vi "04.2 Create Invoke Nodes.vi"() -> ()   [LabVIEW 2019]
uses:
  <vilib>/numeric/Random Number (Range) DBL.vi
panel:
  in  "Stop":bool
  out "Waveform Chart":dbl(graph)
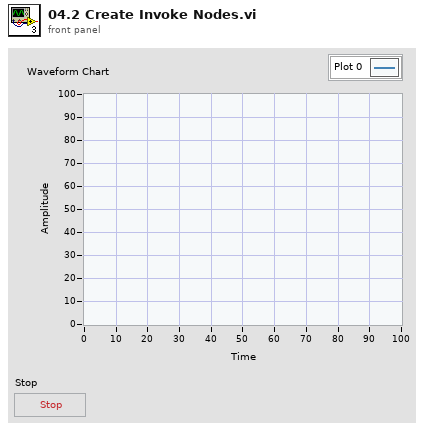
[diagram p1: front panel]
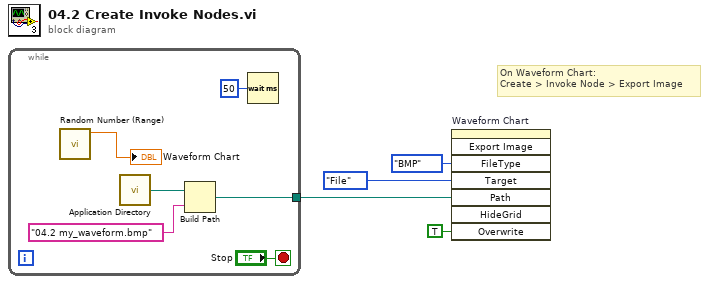
[diagram p0: block diagram]
diagram:
  # "On Waveform Chart:\nCreate > Invoke Node > Export Image"
  n1 = while {
    tunnel: [w6] -> w2
    stop <- "Stop" stop-if-true
    n2 = call-poly <vilib>:"Random Number (Range).vi"() -> ("number"=→"Waveform Chart":dbl)  [unwired: 11 in]
    n3 = call <vilib>:"Application Directory.vi"() -> ("Application Directory"=w8:path)
    n4 = Build Path(base path=w8, name or relative path="04.2 my_waveform.bmp") -> (appended path=w6:path)
    n5 = Wait (ms)(milliseconds to wait=u32 50) -> ()  [unwired: 1 out]
  }
  n6 = invoke on="Waveform Chart" class="WFChart (strict)" method="Export Image"("FileType"=enum32{"BMP", "EPS", "EMF", "PICT"}."BMP" ("File Type"), "Target"=enum32{"File", "Clipboard"}."File", "Path"=w2, "Overwrite"=TRUE ("Always Overwrite")) -> ()  [unwired: 4 in, 8 out]
